vi "Close.vi"(8 "error in":errorcluster, 11 "Humidity Gradient in":refnum<class "Humidity Gradient.lvclass">) -> (0 "error out":errorcluster, 3 "Humidity Gradient out":refnum<class "Humidity Gradient.lvclass">)   [LabVIEW 2023, in "Humidity Gradient.lvclass"]
uses:
  Humidity Gradient.lvclass
  Parents/Gradient/Gradient.lvclass
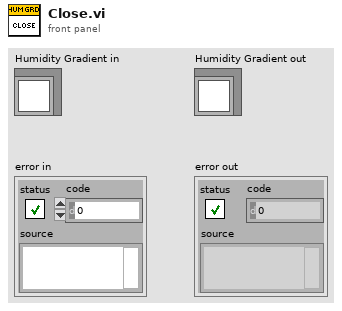
[diagram p1: front panel]
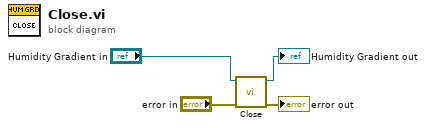
[diagram p0: block diagram]
diagram:
  n1 = call-parent "Close.vi"("error in"="error in", "Gradient in"="Humidity Gradient in") -> ("error out"=→"error out":errorcluster, "Gradient out"=→"Humidity Gradient out":refnum<class "Humidity Gradient.lvclass">)  [unwired: 8 in]
